vi "Picolog Set Sample Rate.vi"(8 "error in (no error)":errorcluster, 9 "Sampling Interval [s]":dbl=0.2 min=0.1 max=100.0 step=0.1 format="%#_13g", 11 "Instrument Handle In":i16) -> (0 "error out":errorcluster, 1 "Actual Sampling Interval [s]":dbl, 3 "Instrument Handle Out":i16)   [LabVIEW 2017]
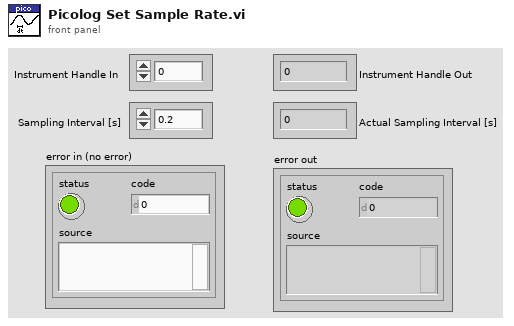
[diagram p1: front panel]
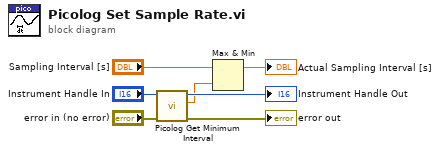
[diagram p0: block diagram]
diagram:
  n1 = call "Picolog Get Minimum Interval.vi"("Error In"="error in (no error)", "Instrument Handle In"="Instrument Handle In") -> ("Error Out"=→"error out":errorcluster, "Minimum Interval [s]"=w2:dbl, "Instrument Handle Out"=→"Instrument Handle Out":i16)  [unwired: 7 in]
  n2 = Max & Min(x="Sampling Interval [s]", y=w2) -> (max(x,y)=→"Actual Sampling Interval [s]":dbl)  [unwired: 1 out]
